vi "Get Relative Time.vi"(7 "Init?":bool, 11 "Time Stamp In":timestamp) -> (1 "dt (ms)":dbl, 2 "Relative System Clock (ms)":dbl, 3 "Time Stamp Out":timestamp)   [LabVIEW 2013, in "PMU Recorder Light.lvlib" / "Statnett C37.118 DLL.lvclass"]
uses:
  Statnett C37.118 DLL.lvclass
  PMU Recorder Light.lvlib
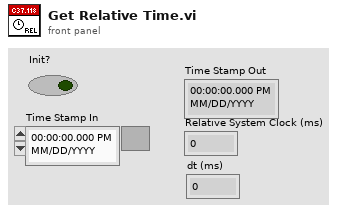
[diagram p1: front panel]
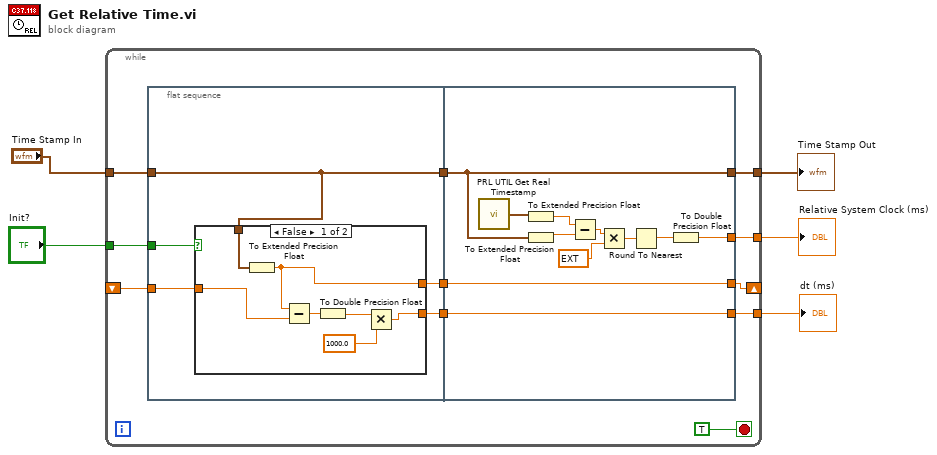
[diagram p0: block diagram]
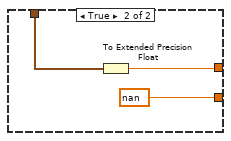
[diagram p2: hidden frame]
diagram:
  n1 = while {
    tunnel: [w15] -> w2
    tunnel: "Init?" -> [w14]
    tunnel: [w13] -> w4
    shift-right: [w10] -> _
    shift-left: _ -> [w12]
    tunnel: [w8] -> w5
    tunnel: "Time Stamp In" -> [w6]
    stop <- TRUE stop-if-true
    n2 = flat-sequence {
      tunnel: [w17] -> w16
      tunnel: w14 -> [w21]
      tunnel: w12 -> [w20]
      tunnel: [w19] -> w11
      tunnel: [w18] -> w9
      tunnel: w6 -> [w17]
      tunnel: w16 -> [w35]
      tunnel: [w36] -> w15
      tunnel: [w35] -> w13
      tunnel: w11 -> [w34]
      tunnel: [w34] -> w10
      tunnel: w9 -> [w33]
      tunnel: [w33] -> w8
      frame #0 {
        n3 = case shown="False" w21 {
          tunnel: w17 -> [w28 w29]
          tunnel: w20 -> [w27 _]
          tunnel: [w26 w30] -> w19
          tunnel: [w23 nan] -> w18
          frame False {
            n4 = To Extended Precision Float(1:w28) -> (0:w26:ext)
            n5 = Subtract(x=w26, y=w27) -> (x-y=w25:ext)
            n6 = To Double Precision Float(number=w25) -> (double precision float=w24:dbl)
            n7 = Multiply(x=w24, y=1000.0) -> (x*y=w23:dbl)
          }
          frame True {
            n8 = To Extended Precision Float(1:w29) -> (0:w30:ext)
          }
        }
      }
      frame #1 {
        n9 = call "PRL UTIL Get Real Timestamp.vi"() -> ("Time Stamp"=w32:timestamp)
        n10 = To Extended Precision Float(1:w32) -> (0:w42:ext)
        n11 = To Extended Precision Float(1:w35) -> (0:w41:ext)
        n12 = Subtract(x=w42, y=w41) -> (x-y=w40:ext)
        n13 = Multiply(x=w40, y=ext 1000.0) -> (x*y=w38:ext)
        n14 = Round To Nearest(number=w38) -> (nearest integer value=w37:ext)
        n15 = To Double Precision Float(number=w37) -> (double precision float=w36:dbl)
      }
    }
  }
  "Time Stamp Out" <- w4
  "Relative System Clock (ms)" <- w2
  "dt (ms)" <- w5
